vi "Fill Line To.vi"(5 "Col":i32, 6 "Attributes":T1, 7 "Row":i32, 8 "error in (no error)":errorcluster, 10 "Char":string, 11 "TermBuffer in":refnum<class "TermBuffer.lvclass">) -> (0 "error out":errorcluster, 3 "TermBuffer out":refnum<class "TermBuffer.lvclass">)   [LabVIEW 2020, in "Terminal.lvlib" / "TermBuffer.lvclass"]
uses:
  TermBuffer.lvclass
  TermBuffer.lvclass/TermBuffer.ctl
  TermLine/TermLine.lvclass
  Text Attributes.ctl
  Terminal.lvlib
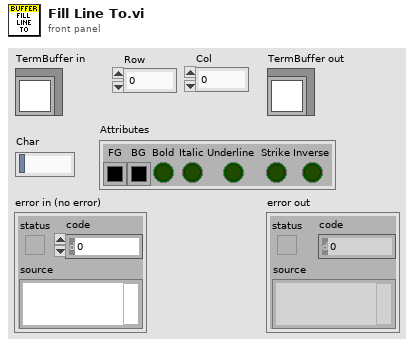
[diagram p1: front panel]
types:
  T1 = typedef "Terminal.lvlib/Text Attributes.ctl" = cluster{"FG":u32, "BG":u32, "Bold":bool, "Italic":bool, "Underline":bool, "Strike":bool, "Inverse":bool}
  T2 = typedef "Terminal.lvlib/TermBuffer.lvclass/Ref Data.ctl" = cluster{"Lines":refnum<class "TermLine.lvclass">[], "Rows":i32, "Cols":i32}
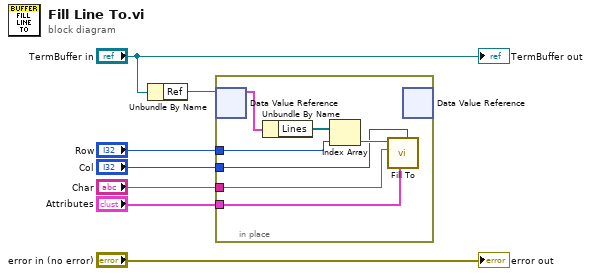
[diagram p0: block diagram]
diagram:
  n1 = Unbundle By Name("TermBuffer in") -> ("Ref"=w6:refnum<data-value>)
  n2 = in-place {
    in-place-border: "Row" -> [w9]
    in-place-border: "Col" -> [w8]
    in-place-border: "Char" -> [w12]
    in-place-border: "Attributes" -> [w11]
    n3 = in-place-dvr #1(w6) -> (w14:T2)  [unwired: 1 out]
    n4 = Unbundle By Name(w14) -> ("Lines"=w13:refnum<class "TermLine.lvclass">[])
    n5 = Index Array(array=w13, index=w9) -> (element=w10:refnum<class "TermLine.lvclass">)
    n6 = call "Fill To.vi"("Col"=w8, "Attributes"=w11, "Char"=w12, "TermLine in"=w10) -> ()  [unwired: 6 in, 2 out]
    n7 = in-place-dvr #1() -> ()  [unwired: 1 in, 2 out]
  }
  "error out" <- "error in (no error)"
  "TermBuffer out" <- "TermBuffer in"
